vi "FPGA main.vi"() -> ()   [LabVIEW 2018]
uses:
  <vilib>/rvi/Emulation/niFpgaGetClockAttributes.vi
  <vilib>/rvi/Emulation/niFpgaSctlEmulationGetInTimedLoop.vi
  <vilib>/rvi/Emulation/niFpgaEmulationReportErrorSimple.vi
  <vilib>/rvi/eio/common/nirviEmuTemplateMethod_errors.vi
  <vilib>/rvi/Emulation/niFpgaCriticalErrorInLSC.vi
  <vilib>/rvi/Emulation/niFpgaProcessEmulError.vi
  <vilib>/eio/EIONode/EIONode.xnode
panel:
  out "Nível Tanque 4":fxp<+/-,16,5>
  out "Nível Tanque 3":fxp<+/-,16,5>
  out "Nível Tanque 2":fxp<+/-,16,5>
  out "Nível Tanque 1":fxp<+/-,16,5>
  in  "Valvula proporcional 2":fxp<+/-,20,5>
  in  "Valvula proporcional 1":fxp<+/-,20,5>
  in  "Temporização FPGA":u32=10000 caption="Tempo de despejo de emergência"
  in  "Bomba 2":fxp<+/-,20,5>
  in  "Bomba 1":fxp<+/-,20,5>
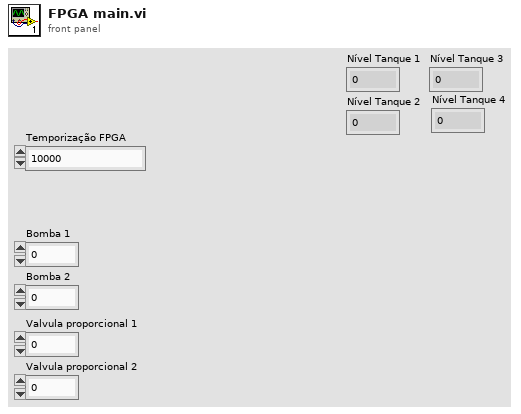
[diagram p1: front panel]
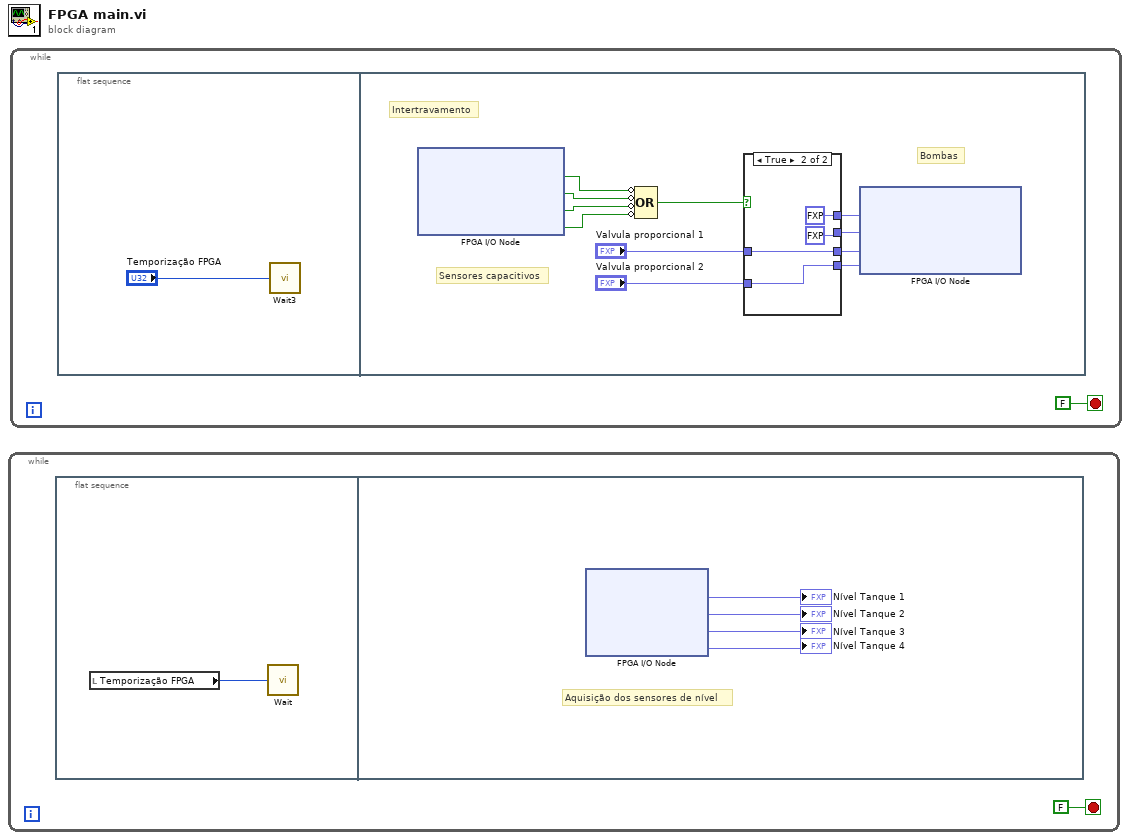
[diagram p0: block diagram]
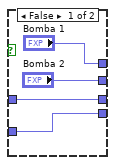
[diagram p2: hidden frame]
diagram:
  n1 = while {
    stop <- FALSE stop-if-true
    n2 = flat-sequence {
      frame #0 {
        n3 = local read "Temporização FPGA"() -> (w2:u32)
        n4 = call "Wait"("Count(mSec)"=w2) -> ()  [unwired: 1 out]
      }
      frame #1 {
        # "Aquisição dos sensores de nível"
        n5 = xnode "FPGA I/O Node"() -> ("Nível Tanque 1"=→"Nível Tanque 1":fxp<+/-,16,5>, "Nível Tanque 2"=→"Nível Tanque 2":fxp<+/-,16,5>, "Nível Tanque 3"=→"Nível Tanque 3":fxp<+/-,16,5>, "Nível Tanque 4"=→"Nível Tanque 4":fxp<+/-,16,5>)  [unwired: 4 in, 4 out]
      }
    }
  }
  n6 = while {
    stop <- FALSE stop-if-true
    n7 = flat-sequence {
      frame #0 {
        n8 = call "Wait3"("Count(mSec)"="Temporização FPGA") -> ()  [unwired: 1 out]
      }
      frame #1 {
        # "Bombas"
        # "Sensores capacitivos"
        # "Intertravamento"
        n9 = xnode "FPGA I/O Node"() -> ("Sensor Capacitivo 1"=w16:bool, "Sensor Capacitivo 2"=w15:bool, "Sensor Capacitivo 3"=w13:bool, "Sensor Capacitivo 4"=w14:bool)  [unwired: 4 in, 4 out]
        n10 = Compound Arithmetic op=OR(invert w16, invert w15, invert w13, invert w14) -> (w17:bool)
        n11 = case shown="True" w17 {
          tunnel: ["Bomba 1" fxp<+/-,20,5> 0.0 ("Saídas Analógicas/AO0")] -> w12
          tunnel: ["Bomba 2" fxp<+/-,20,5> 0.0 ("Saídas Analógicas/AO1")] -> w11
          tunnel: [w21 w25] -> w10
          tunnel: "Valvula proporcional 1" -> [w21 w25]
          tunnel: [w20 w24] -> w9
          tunnel: "Valvula proporcional 2" -> [w20 w24]
          frame False {
          }
          frame True {
          }
        }
        n12 = xnode "FPGA I/O Node"("Bomba 1"=w12, "Bomba 2"=w11, "Válvula Proporcional 1"=w10, "Válvula Proporcional 2"=w9) -> ()  [unwired: 4 in, 4 out]
      }
    }
  }
